vi "DefaultValueClassPath--Constant.vi"() -> (3 "DefaultValueClassPath":string)   [LabVIEW 2021, in "IconEditorInterface.lvlib" / "IconEditorInterface.lvclass"]
uses:
  <resource>/plugins/NIIconEditor/UI/Interface class/IconEditorInterface.lvclass
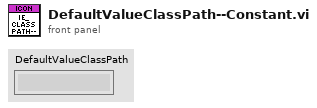
[diagram p1: front panel]
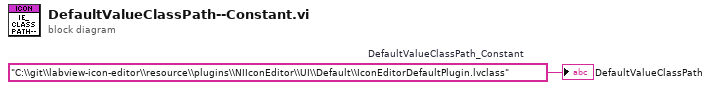
[diagram p0: block diagram]
diagram:
  w1 = "C:\\git\\labview-icon-editor\\resource\\plugins\\NIIconEditor\\UI\\Default\\IconEditorDefaultPlugin.lvclass"  # DefaultValueClassPath_Constant
  "DefaultValueClassPath" <- w1
